vi "Tosca-Monitor Transitions.vi"(0 "Flow Element":refnum<class "State.lvclass">, 1 "Decision state":string, 2 "Message":refnum<queue>, 7 "State":i32, 9 "Trial type":T1, 11 "error in":errorcluster) -> (4 "Result String":string, 8 "Next":i32, 10 "End on rep":bool, 12 "Trxn":i32, 13 "Result":T2, 14 "named result":bool, 15 "error out":errorcluster)   [LabVIEW 2020]
uses:
  Typedefs/Tosca-Trial Result Enum.ctl
  IPC VIs/Tosca-Message.ctl
  IPC VIs/Tosca-Message Action.ctl
  Classes/State/State.lvclass
  Typedefs/Tosca-Event Type.ctl
  Typedefs/Tosca-Transition Progress.ctl
  Typedefs/Tosca-TTL Event State.ctl
  Classes/State/State.lvclass/State.ctl
  Classes/Termination/Termination.lvclass/Termination.ctl
  Classes/Timeout/Timeout.lvclass/Timeout.ctl
  Classes/Termination/Read TTL.vi
  Classes/Timeout/Read TTL.vi
  Classes/Timeout/Read Next.vi
  Classes/Timeout/Read Result.vi
  Classes/State/Read Name.vi
  Classes/State/Read script.vi
  TTL VIs/Control Classes/Base Class/TTLController.lvclass
  Classes/Timeout/Timeout.lvclass
  Classes/Termination/Termination.lvclass
panel:
  in  "Poll Interval (ms)":u32=10
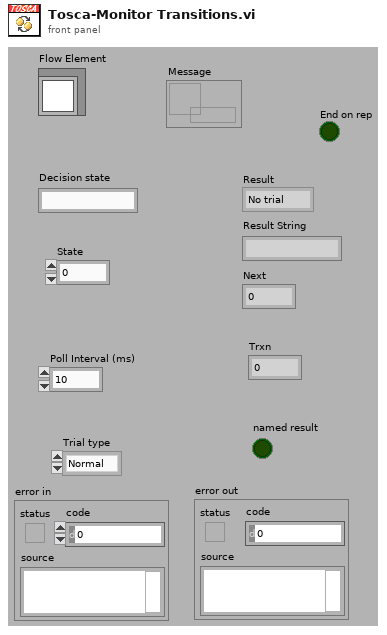
[diagram p1: front panel]
types:
  T1 = typedef "Tosca-Event Type.ctl" = enum16{"Normal", "CS+", "CS-"}
  T2 = typedef "Tosca-Trial Result Enum.ctl" = enum16{"No trial", "Go", "No go", "Error", "Abort"}
  T3 = typedef "Tosca-TTL Event State.ctl" = cluster{"N":i32, "Tlast":dbl, "value":bool}
  T4 = typedef "Tosca-Transition Progress.ctl" = cluster{"Tstart":u32, "Tnow":u32, "Tend":dbl, "Next state":i32, "Cause":string, "Result":T2, "Events":cluster{"Value":bool, "Time":u32}[], "end on rep":bool, "Trxn":i32}
  T5 = typedef "Tosca-Message Action.ctl" = enum16{"None", "Update", "Events", "Timeout", "Error", "Abort"}
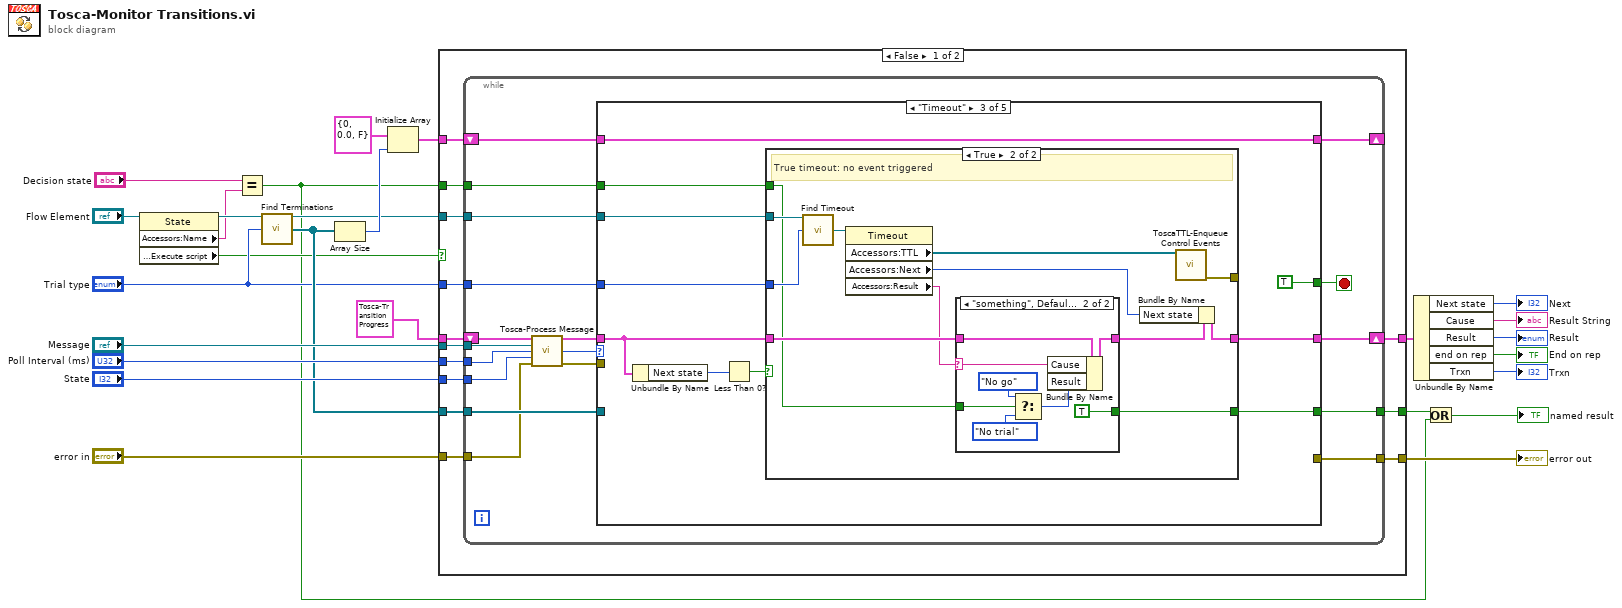
[diagram p0: block diagram]
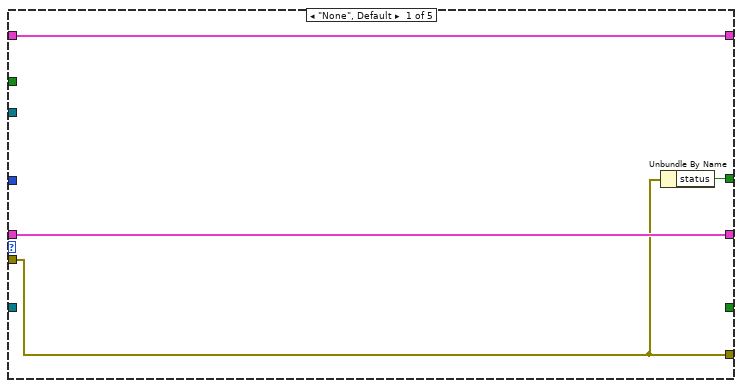
[diagram p2: hidden frame]
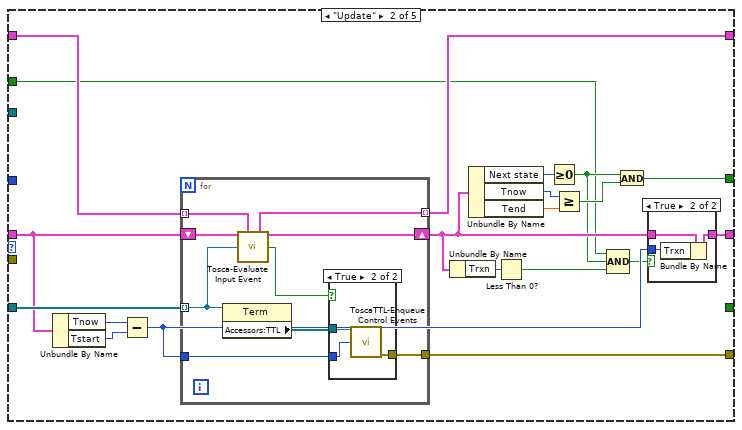
[diagram p3: hidden frame]
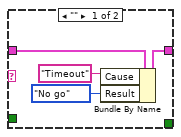
[diagram p7: hidden frame]
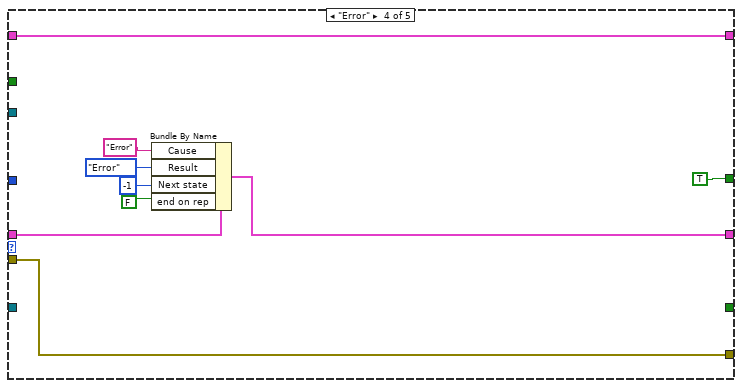
[diagram p8: hidden frame]
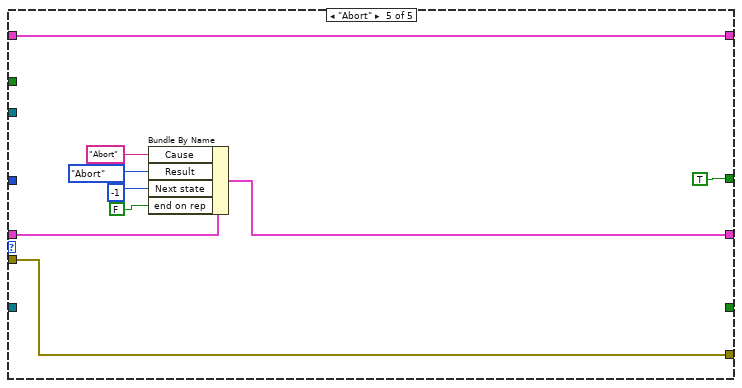
[diagram p9: hidden frame]
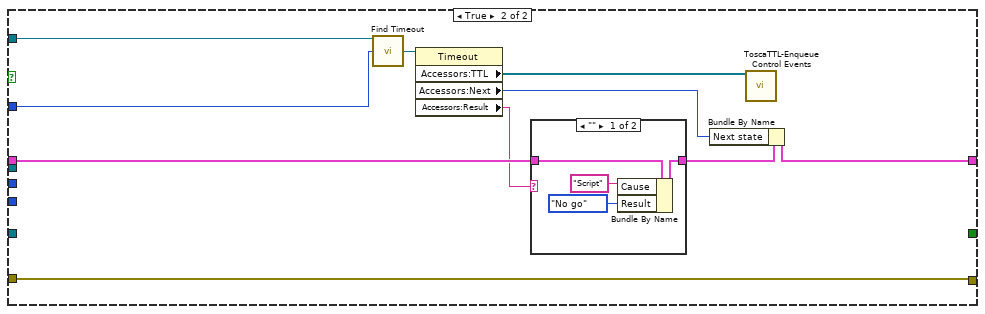
[diagram p10: hidden frame]
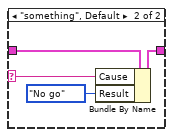
[diagram p11: hidden frame]
diagram:
  n1 = property class="State"(reference="Flow Element") -> (reference out=w7:refnum<class "State.lvclass">, "Accessors:Name"=w6:string, "Accessors:Execute script"=w4:bool)  [unwired: 1 in, 1 out]
  n2 = Equal?(x="Decision state", y=w6) -> (x = y?=w1:bool)
  n3 = call "Find Terminations.vi"("State in"=w7, "Type"="Trial type") -> ("State thru"=w10:refnum<class "State.lvclass">, "Terminations"=w11:refnum<class "Termination.lvclass">[])  [unwired: 11 in, 1 out]
  n4 = Array Size(array=w11) -> (size(s)=w14:i32)
  n5 = Initialize Array(T3 {"N"=0, "Tlast"=0.0, "value"=FALSE} ("State"), w14) -> (w13:T3[])
  n6 = case shown="False" w4 {
    tunnel: "error in" -> [w39 w156]
    tunnel: [w38 w156] -> w25
    tunnel: "Message" -> [w37 _]
    tunnel: "Poll Interval (ms)" -> [w36 _]
    tunnel: "State" -> [w35 _]
    tunnel: T4 {"Tstart"=0, "Tnow"=0, "Tend"=0.0, "Next state"=-1, "Cause"="Timeout", "Result"=enum."No trial", "Events"=[], "end on rep"=FALSE, "Trxn"=-1} ("Progress") -> [w34 w160]
    tunnel: [w33 w159] -> w20
    tunnel: w13 -> [w32 _]
    tunnel: w11 -> [w31 _]
    tunnel: w10 -> [w30 w158]
    tunnel: "Trial type" -> [w29 w157]
    tunnel: w1 -> [w28 _]
    tunnel: [w27 _] -> w3
    frame False {
      n7 = while {
        tunnel: w39 -> [w47]
        tunnel: [w56] -> w38
        tunnel: w31 -> [w55]
        tunnel: w37 -> [w54]
        tunnel: w36 -> [w53]
        tunnel: w35 -> [w52]
        shift-right: [w46] -> w33
        shift-left: w34 -> [w51]
        shift-right: [w44] -> _
        shift-left: w32 -> [w45]
        tunnel: w30 -> [w43]
        tunnel: w29 -> [w42]
        tunnel: w28 -> [w41]
        tunnel: [w40] -> w27
        stop <- w57 stop-if-true
        n8 = call "Tosca-Process Message.vi"("Progress In"=w51, "Message"=w54, "timeout in ms"=w53, "State"=w52, "error in (no error)"=w47) -> ("Progress Out"=w49:T4, "Action"=w50:T5, "error out"=w48:errorcluster)  [unwired: 8 in]
        n9 = case shown="\"Timeout\"" w50 {
          tunnel: w55 -> [_ w81 _ _ _]
          tunnel: [w60 w75 _ w135 w144] -> w56
          tunnel: [w59 w76 TRUE TRUE TRUE] -> w57
          tunnel: w49 -> [w61 w68 w104 w140 w149]
          tunnel: [w61 w66 w103 w136 w145] -> w46
          tunnel: w48 -> [w60 _ _ w135 w144]
          tunnel: w45 -> [w58 w74 w102 w133 w142]
          tunnel: [w58 w73 w102 w133 w142] -> w44
          tunnel: w43 -> [_ _ w101 _ _]
          tunnel: w42 -> [_ _ w100 _ _]
          tunnel: w41 -> [_ w62 w98 _ _]
          tunnel: [_ _ w99 _ _] -> w40
          frame "None", Default {
            n10 = Unbundle By Name(w60) -> ("status"=w59:bool)
          }
          frame "Update" {
            n11 = Unbundle By Name(w68) -> ("Tnow"=w72:u32, "Tstart"=w71:u32)
            n12 = Subtract(x=w72, y=w71) -> (x-y=w65:u32)
            n13 = for {
              tunnel: w81 -> [w86] mode=indexing
              shift-right: [w93] -> w67
              shift-left: w68 -> [w94]
              tunnel: w74 -> [w92] mode=indexing
              tunnel: [w91] -> w73 mode=indexing
              tunnel: [w90] -> w75
              tunnel: w65 -> [w88]
              n14 = property class="Term"(reference=w86) -> ("Accessors:TTL"=w87:refnum<class "TTLController.lvclass">[])  [unwired: 1 in, 2 out]
              n15 = call "Tosca-Evaluate Input Event.vi"("Progress In"=w94, "Event state in"=w92, "Term"=w86) -> ("Event state out"=w91:T3, "Progress Out"=w93:T4, "TTL condition true"=w89:bool)  [unwired: 10 in]
              n16 = case shown="True" w89 {
                tunnel: w87 -> [_ w97]
                tunnel: [_ w96] -> w90
                tunnel: w88 -> [_ w95]
                frame False {
                }
                frame True {
                  n17 = call "ToscaTTL-Enqueue Control Events.vi"("TTL"=w97, "Rxn time"=w95) -> ("error out"=w96:errorcluster)  [unwired: 13 in]
                }
              }
            }
            n18 = Unbundle By Name(w67) -> ("Trxn"=w70:i32)
            n19 = Unbundle By Name(w67) -> ("Next state"=w80:i32, "Tnow"=w79:u32, "Tend"=w78:dbl)
            n20 = Less Than 0?(x=w70) -> (x < 0?=w69:bool)
            n21 = Greater Or Equal To 0?(x=w80) -> (x >= 0?=w63:bool)
            n22 = Greater Or Equal?(x=w79, y=w78) -> (x >= y?=w77:bool)
            n23 = Compound Arithmetic op=AND(w62, w63, w69) -> (w64:bool)
            n24 = And(x=w63, y=w77) -> (x .and. y?=w76:bool)
            n25 = case shown="True" w64 {
              tunnel: w67 -> [w82 w83]
              tunnel: [w82 w85] -> w66
              tunnel: w65 -> [_ w84]
              frame False {
              }
              frame True {
                n26 = Bundle By Name(cluster=w83, "Trxn"=w84) -> (w85:T4)
              }
            }
          }
          frame "Timeout" {
            n27 = Unbundle By Name(w104) -> ("Next state"=w106:i32)
            n28 = Less Than 0?(x=w106) -> (x < 0?=w105:bool)
            n29 = case shown="True" w105 {
              tunnel: w104 -> [w108 w119]
              tunnel: [w108 w118] -> w103
              tunnel: [_ w117] -> _
              tunnel: w101 -> [_ w116]
              tunnel: w100 -> [_ w115]
              tunnel: [_ w110] -> w99
              tunnel: w98 -> [_ w109]
              frame False {
                # "Input event triggered, but with delayed transition"
              }
              frame True {
                # "True timeout: no event triggered"
                n30 = call "Find Timeout.vi"("State in"=w116, "Type"=w115) -> ("Timeout"=w114:refnum<class "Timeout.lvclass">)  [unwired: 11 in, 2 out]
                n31 = property class="Timeout"(reference=w114) -> ("Accessors:TTL"=w113:refnum<class "TTLController.lvclass">[], "Accessors:Next"=w111:i32, "Accessors:Result"=w112:string)  [unwired: 1 in, 2 out]
                n32 = case shown="\"something\", Default" w112 {
                  selector: w112 -> [_ w130]
                  tunnel: [w123 w131] -> w120
                  tunnel: w119 -> [w124 w132]
                  tunnel: [_ TRUE] -> w110
                  tunnel: w109 -> [_ w128]
                  frame "" {
                    # "Target state?"
                    n33 = Bundle By Name(cluster=w124, "Cause"="Timeout", "Result"=Tosca-Trial_Result_Enum."No go") -> (w123:T4)
                  }
                  frame "something", Default {
                    # "Target state?"
                    n34 = Select(t=Tosca-Trial_Result_Enum."No go" ("Result"), s=w128, f=Tosca-Trial_Result_Enum."No trial" ("Result")) -> (s? t:f=w126:T2)
                    n35 = Bundle By Name(cluster=w132, "Cause"=w130, "Result"=w126) -> (w131:T4)
                  }
                }
                n36 = Bundle By Name(cluster=w120, "Next state"=w111) -> (w118:T4)
                n37 = call "ToscaTTL-Enqueue Control Events.vi"("TTL"=w113) -> ("error out"=w117:errorcluster)  [unwired: 14 in]
              }
            }
          }
          frame "Error" {
            n38 = Bundle By Name(cluster=w140, "Cause"="Error", "Result"=Tosca-Trial_Result_Enum."Error", "Next state"=-1, "end on rep"=FALSE) -> (w136:T4)
          }
          frame "Abort" {
            n39 = Bundle By Name(cluster=w149, "Cause"="Abort", "Result"=Tosca-Trial_Result_Enum."Abort", "Next state"=-1, "end on rep"=FALSE) -> (w145:T4)
          }
        }
      }
    }
    frame True {
      n40 = call "Find Timeout.vi"("State in"=w158, "Type"=w157) -> ("Timeout"=w154:refnum<class "Timeout.lvclass">)  [unwired: 11 in, 2 out]
      n41 = property class="Timeout"(reference=w154) -> ("Accessors:TTL"=w153:refnum<class "TTLController.lvclass">[], "Accessors:Next"=w151:i32, "Accessors:Result"=w152:string)  [unwired: 1 in, 2 out]
      n42 = case shown="\"\"" w152 {
        selector: w152 -> [_ w165]
        tunnel: [w163 w167] -> w155
        tunnel: w160 -> [w164 w168]
        frame "" {
          # "Target state?"
          n43 = Bundle By Name(cluster=w164, "Cause"="Script", "Result"=Tosca-Trial_Result_Enum."No go") -> (w163:T4)
        }
        frame "something", Default {
          # "Target state?"
          n44 = Bundle By Name(cluster=w168, "Cause"=w165, "Result"=Tosca-Trial_Result_Enum."No go") -> (w167:T4)
        }
      }
      n45 = Bundle By Name(cluster=w155, "Next state"=w151) -> (w159:T4)
      n46 = call "ToscaTTL-Enqueue Control Events.vi"("TTL"=w153) -> ()  [unwired: 14 in, 1 out]
    }
  }
  "error out" <- w25
  n47 = Unbundle By Name(w20) -> ("Next state"=→"Next":i32, "Cause"=→"Result String":string, "Result"=→"Result":T2, "end on rep"=→"End on rep":bool, "Trxn"=→"Trxn":i32)
  n48 = Or(x=w3, y=w1) -> (x .or. y?=→"named result":bool)
